vi "PassInterception.vi"(6 "Ally?":bool, 8 "error in (no error)":errorcluster, 9 "Point":dbl[](array[numeric]), 10 "GameRef":refnum<data-value>, 11 "BallInterception in":refnum<class "BallInterception.lvclass">) -> (0 "error out":errorcluster, 2 "Evaluation":dbl, 3 "BallInterception out":refnum<class "BallInterception.lvclass">)   [LabVIEW 2023, in "BallInterception.lvclass"]
uses:
  BallInterception.lvclass
  Game_class/Game.lvclass
  Game_class/Game.lvclass/Game.ctl
  Referee_class/Referee.lvclass/Referee.ctl
  Team_class/Team.lvclass/Team.ctl
  Object_class/Object.lvclass/Object.ctl
  Robot_class/Robot.lvclass/Robot.ctl
  <vilib>/Analysis/coordinate.llb/2D Cartesian Coordinate Shift (Scalar).vi
  <vilib>/Analysis/coordinate.llb/2D Cartesian Coordinate Rotation (Scalar).vi
  Robot_class/Read id.vi
  Object_class/Read position(x,y).vi
  Game_class/Read Referee.vi
  Game_class/Read EnemyRef.vi
  Game_class/Read BallRef.vi
  Game_class/Read AllyRef.vi
  Team_class/Read RobotRef.vi
  Referee_class/Read enemy_goalie_id.vi
  Referee_class/Read our_goalie_id.vi
  Ally_class/Ally.lvclass
  C:/Users/ebert/Documents/codes/SSL/repo/SSL_AI/Team_class/Team.lvclass
  Ball_class/Ball.lvclass
  C:/Users/ebert/Documents/codes/SSL/repo/SSL_AI/Object_class/Object.lvclass
  Enemy_class/Enemy.lvclass
  Robot_class/Robot.lvclass
  Referee_class/Referee.lvclass
  <vilib>/Analysis/NI_AALPro.lvlib
  Utilities_class/Utilities.lvclass
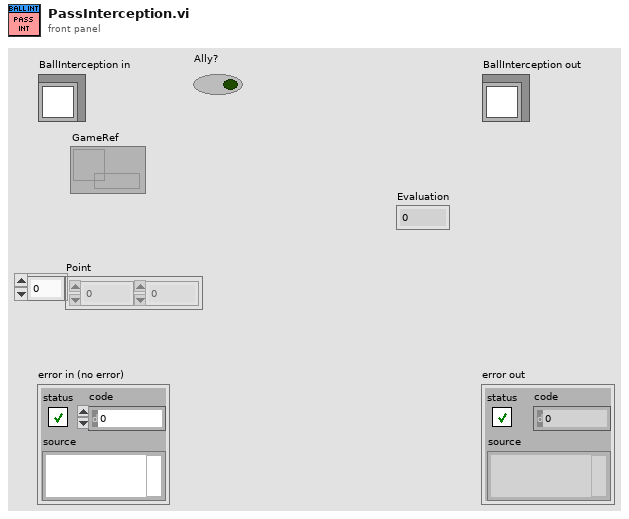
[diagram p1: front panel]
types:
  T1 = typedef "STPParameters.ctl" = cluster{"Skills":T2, "TestSkill":T4, "Events":cluster{"distanceToBallPossession":dbl, "timeForPossessionThreshold":dbl}, "Criteria":cluster{"OpenAngleToGoal":cluster{"minAngle":dbl, "maxAngle":dbl, "minEvaluation":dbl}, "PassDistance":cluster{"maxDistance":dbl, "minDistance":dbl}, "ShotInterception":cluster{"shotSpeed":dbl, "minEnemySpeed":dbl, "minEvaluation":dbl, "maxEnemySpeed":dbl}, "OneTouchShot":cluster{"MaxAngle":dbl, "minEvaluation":dbl}, "PassInterception":cluster{"minEnemySpeed":dbl, "maxEnemySpeed":dbl, "chipPassDistance":dbl, "chipPassEval":dbl, "minEvaluation":dbl}}, "minPassSpeed":dbl, "maxPassSpeed":dbl, "AllyTeamIds":T5[]}
  T2 = typedef "Skills.ctl" = cluster{"CirculateBall":T3, "ProtectBall":cluster{"DistanceFromBall":dbl}}
  T3 = typedef "CIrculateSkillParameters.ctl" = cluster{"rotationAngle":dbl, "velocityFactor":dbl, "OrientationFactor":dbl}
  T4 = typedef "TestSkills.ctl" = enum16{"AlignSkill", "PassSkill", "CirculateBall", "OneTouchShotSkill", "KickToSkill_v2", "ShootSkill", "InterceptBall", "Exit", "GoToSkill_v2"}
  T5 = typedef "AllyTeam.ctl" = enum16{"Keeper", "Defender", "Attacker"}
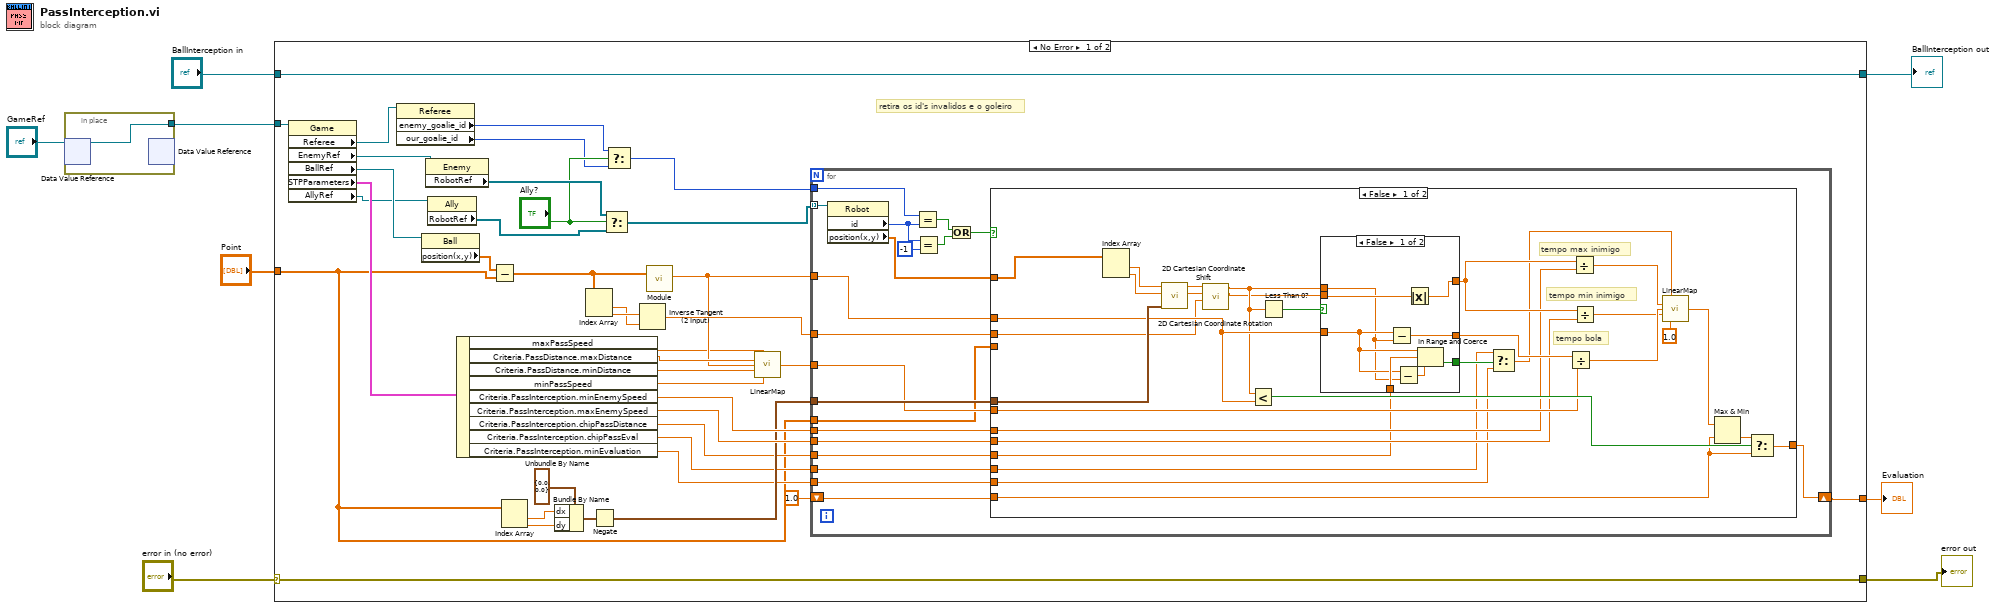
[diagram p0: block diagram]
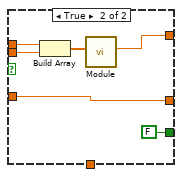
[diagram p2: hidden frame]
diagram:
  n1 = in-place {
    in-place-border: [w9] -> w1
    n2 = in-place-dvr #1("GameRef") -> (w9:refnum<class "Game.lvclass">)  [unwired: 1 out]
    n3 = in-place-dvr #1() -> ()  [unwired: 1 in, 2 out]
  }
  n4 = case shown="No Error" "error in (no error)" {
    selector: "error in (no error)" -> [w48 w115]
    tunnel: [w48 w115] -> w3
    tunnel: "BallInterception in" -> [w47 w114]
    tunnel: [w47 w114] -> w5
    tunnel: w1 -> [w46 _]
    tunnel: "Point" -> [w19 _]
    tunnel: [w29 _] -> w7
    frame No Error {
      # "retira os id's invalidos e o goleiro"
      n5 = property class="Game"(reference=w46) -> ("Referee"=w44:refnum<class "Referee.lvclass">, "EnemyRef"=w45:refnum<class "Enemy.lvclass">, "BallRef"=w43:refnum<class "Ball.lvclass">, "STPParameters"=w35:T1, "AllyRef"=w11:refnum<class "Ally.lvclass">)  [unwired: 1 in, 2 out]
      n6 = property class="Referee"(reference=w44) -> ("enemy_goalie_id"=w14:i32, "our_goalie_id"=w12:i32)  [unwired: 1 in, 2 out]
      n7 = property class="Ball"(reference=w43) -> ("position(x,y)"=w18:dbl[])  [unwired: 1 in, 2 out]
      n8 = property class="Enemy"(reference=w45) -> ("RobotRef"=w17:refnum<class "Robot.lvclass">[])  [unwired: 1 in, 2 out]
      n9 = property class="Ally"(reference=w11) -> ("RobotRef"=w10:refnum<class "Robot.lvclass">[])  [unwired: 1 in, 2 out]
      n10 = Unbundle By Name(w35) -> ("maxPassSpeed"=w27:dbl, "Criteria.PassDistance.maxDistance"=w34:dbl, "Criteria.PassDistance.minDistance"=w33:dbl, "minPassSpeed"=w28:dbl, "Criteria.PassInterception.minEnemySpeed"=w26:dbl, "Criteria.PassInterception.maxEnemySpeed"=w25:dbl, "Criteria.PassInterception.chipPassDistance"=w22:dbl, "Criteria.PassInterception.chipPassEval"=w21:dbl, "Criteria.PassInterception.minEvaluation"=w20:dbl)
      n11 = Subtract(x=w18, y=w19) -> (x-y=w36:dbl[])
      n12 = Index Array(array=w19) -> (element #1=w38:dbl, element #2=w37:dbl)  [unwired: 2 in]
      n13 = Bundle By Name(cluster=cluster{"dx":dbl, "dy":dbl} {"dx"=0.0, "dy"=0.0} ("shift"), "dx"=w38, "dy"=w37) -> (w24:cluster{"dx":dbl, "dy":dbl})
      n14 = Index Array(array=w36) -> (element #1=w41:dbl, element #2=w42:dbl)  [unwired: 2 in]
      n15 = Negate(x=w24) -> (-x=w23:cluster{"dx":dbl, "dy":dbl})
      n16 = Select(t=w17, s="Ally?", f=w10) -> (s? t:f=w16:refnum<class "Robot.lvclass">[])
      n17 = Select(t=w14, s="Ally?", f=w12) -> (s? t:f=w13:i32)
      n18 = Inverse Tangent (2 Input)(1:w41, 2:w42) -> (0:w40:dbl)
      n19 = call "Module.vi"("2D vector"=w36) -> ("Modulo"=w32:dbl)  [unwired: 8 in, 2 out]
      n20 = call "LinearMap.vi"("MaxY"=w27, "MaxX"=w34, "X"=w32, "MinX"=w33, "MinY"=w28) -> ("Y"=w31:dbl)  [unwired: 8 in, 2 out]
      n21 = for {
        tunnel: w16 -> [w67] mode=indexing
        tunnel: w13 -> [w49]
        tunnel: w40 -> [w62]
        tunnel: w23 -> [w60]
        tunnel: w32 -> [w59]
        tunnel: w31 -> [w58]
        shift-right: [w56] -> w29
        shift-left: 1.0 ("Numeric") -> [w57]
        tunnel: w19 -> [w55]
        tunnel: w26 -> [w54]
        tunnel: w25 -> [w53]
        tunnel: w22 -> [w52]
        tunnel: w21 -> [w51]
        tunnel: w20 -> [w50]
        n22 = property class="Robot"(reference=w67) -> ("id"=w66:i32, "position(x,y)"=w61:dbl[])  [unwired: 1 in, 2 out]
        n23 = Equal?(x=w49, y=w66) -> (x = y?=w64:bool)
        n24 = Equal?(x=w66, y=-1) -> (x = y?=w63:bool)
        n25 = Or(x=w64, y=w63) -> (x .or. y?=w68:bool)
        n26 = case shown="False" w68 {
          tunnel: w62 -> [w80 _]
          tunnel: w61 -> [w94 _]
          tunnel: w60 -> [w98 _]
          tunnel: w59 -> [w89 _]
          tunnel: w58 -> [w90 _]
          tunnel: w57 -> [w81 w113]
          tunnel: [w95 w113] -> w56
          tunnel: w55 -> [_ _]
          tunnel: w54 -> [w87 _]
          tunnel: w53 -> [w86 _]
          tunnel: w52 -> [w73 _]
          tunnel: w51 -> [w70 _]
          tunnel: w50 -> [w69 _]
          frame False {
            # "tempo bola"
            # "tempo min inimigo"
            # "tempo max inimigo"
            n27 = Index Array(array=w94) -> (element #1=w79:dbl, element #2=w78:dbl)  [unwired: 2 in]
            n28 = call-poly <vilib>:"2D Cartesian Coordinate Shift.vi"("shift"=w98, "y"=w78, "x"=w79) -> ("y out"=w76:dbl, "x out"=w77:dbl)  [unwired: 6 in, 1 out]
            n29 = call-poly <vilib>:"2D Cartesian Coordinate Rotation.vi"("theta"=w80, "y"=w76, "x"=w77) -> ("y out"=w74:dbl, "x out"=w75:dbl)  [unwired: 6 in, 1 out]
            n30 = Less?(x=w75, y=w89) -> (x < y?=w96:bool)
            n31 = Less Than 0?(x=w75) -> (x < 0?=w97:bool)
            n32 = case shown="False" w97 {
              tunnel: w75 -> [w99 w110]
              tunnel: w74 -> [w105 w108]
              tunnel: [w104 w112] -> w91
              tunnel: w89 -> [w101 w111]
              tunnel: [w106 w111] -> w88
              tunnel: w73 -> [w102 _]
              tunnel: [w100 FALSE] -> w71
              frame False {
                n33 = Subtract(x=w101, y=w99) -> (x-y=w106:dbl)
                n34 = Subtract(x=w101, y=w99) -> (x-y=w103:dbl)
                n35 = Absolute Value(x=w105) -> (abs(x)=w104:dbl)
                n36 = In Range and Coerce(upper limit=w101, x=w102, lower limit=w103) -> (In Range?=w100:bool)  [unwired: 1 out]
              }
              frame True {
                n37 = Build Array(w110, w108) -> (w109:dbl[])
                n38 = call "Module.vi"("2D vector"=w109) -> ("Modulo"=w112:dbl)  [unwired: 8 in, 2 out]
              }
            }
            n39 = Select(t=w70, s=w71, f=w69) -> (s? t:f=w72:dbl)
            n40 = Divide(x=w88, y=w90) -> (x/y=w93:dbl)
            n41 = Divide(x=w91, y=w87) -> (x/y=w85:dbl)
            n42 = Divide(x=w91, y=w86) -> (x/y=w84:dbl)
            n43 = call "LinearMap.vi"("MaxY"=w72, "MaxX"=w85, "X"=w93, "MinX"=w84, "MinY"=1.0) -> ("Y"=w83:dbl)  [unwired: 8 in, 2 out]
            n44 = Max & Min(x=w83, y=w81) -> (min(x,y)=w82:dbl)  [unwired: 1 out]
            n45 = Select(t=w82, s=w96, f=w81) -> (s? t:f=w95:dbl)
          }
          frame True {
          }
        }
      }
    }
    frame Error {
    }
  }
  "error out" <- w3
  "BallInterception out" <- w5
  "Evaluation" <- w7
